vi "PrintVolt (SubVI).vi"(11 "Protocol 2":string[][](table)=[["11.02.26 11:54:00", "3.0012e-3", "3.0012e-3", "125,65", "125,65", "1 В", "1 В"], ["", "", "", "", "", "", ""]]) -> ()   [LabVIEW 2017]
uses:
  <vilib>/Utility/file.llb/Write Delimited Spreadsheet (string).vi
panel:
  out "error out 2":errorcluster caption="error out"
  in  "delimiter (\\t)":string="\t"
  in  "Discription":string[](array[string])=["Время", "Uскз А, В", "Uскз B, В", "Fа, кГц", "Fb, кГц", "Диап. A", "Диап. B", "Прим."]
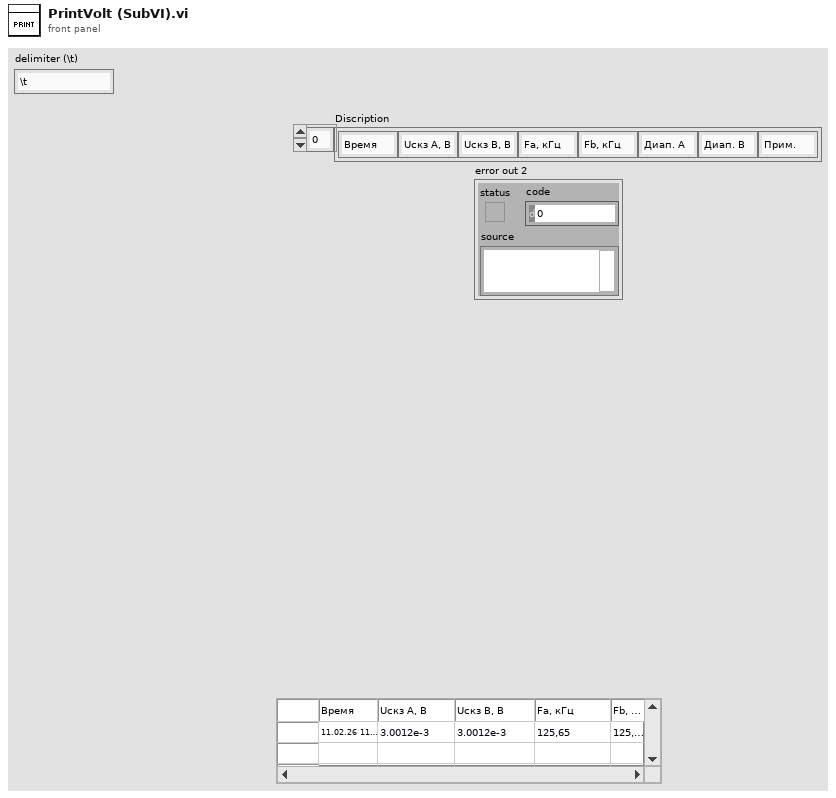
[diagram p1: front panel]
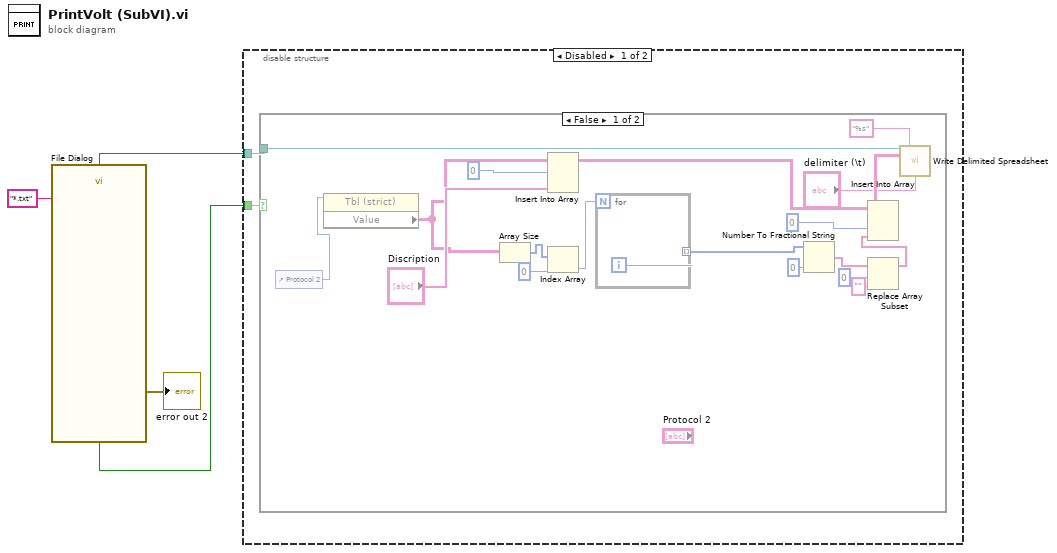
[diagram p0: block diagram]
diagram:
  n1 = call "File Dialog"("pattern (all files)"="*.txt") -> ("selected path"=w4:path, "cancelled"=w3:bool, "error out"=→"error out 2":errorcluster)  [unwired: 11 in, 1 out]
  n2 = disable-structure shown="Disabled" {
    disable-tunnel: w4 -> [w6 _]
    disable-tunnel: w3 -> [w5 _]
    frame Disabled {
      n3 = case shown="False" w5 {
        tunnel: w6 -> [w25 _]
        frame False {
          n4 = control-ref of="Protocol 2"() -> (w7:refnum<vi>)
          n5 = property class="Tbl (strict)"(reference=w7) -> ("Value"=w8:string[][])  [unwired: 1 in, 2 out]
          n6 = Array Size(array=w8) -> (size(s)=w22:i32[])
          n7 = Insert Into Array(array=w8, index (row)=0, new element="Discription") -> (w19:string[][])  [unwired: 1 in]
          n8 = Index Array(array=w22, index=0) -> (element=w20:i32)
          n9 = for {
            N: w20 -> [_]
            tunnel: [w26] -> w16 mode=indexing
            i -> [w26]
          }
          n10 = Number To Fractional String(number=w16, precision (6)=i16 0) -> (F-format string=w14:string[])  [unwired: 2 in]
          n11 = Replace Array Subset(array=w14, new element="" ("new element/subarray"), index=0) -> (w13:string[])
          n12 = Insert Into Array(array=w19, index (col)=0 ("disabled index (col)"), new element=w13) -> (w17:string[][])  [unwired: 1 in]
          n13 = call-poly <vilib>:"Write Delimited Spreadsheet.vi"("file path (dialog if empty)"=w25, "format (%s)"="%s", "2D data"=w17, "delimiter (\\t)"="delimiter (\\t)") -> ()  [unwired: 10 in, 2 out]
        }
        frame True {
        }
      }
    }
    frame Enabled {
    }
  }
